vi "Write output L.vi"(10 "output L":dbl, 11 "PID_OL_AM in":refnum<class "PID_OL_AM.lvclass">) -> (3 "PID_OL_AM out":refnum<class "PID_OL_AM.lvclass">)   [LabVIEW 2019, in "control.lvlib" / "PID_OL_AM.lvclass"]
uses:
  PID_OL_AM.lvclass
  PID_OL_AM.lvclass/PID_OL_AM.ctl
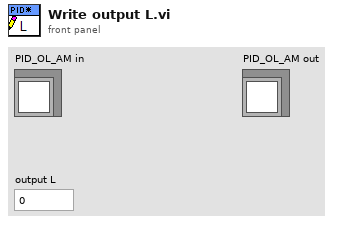
[diagram p1: front panel]
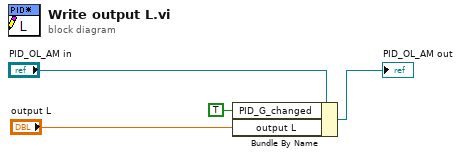
[diagram p0: block diagram]
diagram:
  n1 = Bundle By Name(cluster="PID_OL_AM in", "PID_G_changed"=TRUE, "output L"="output L") -> (→"PID_OL_AM out":refnum<class "PID_OL_AM.lvclass">)
